vi "User Name or Public.vi"() -> ()   [LabVIEW 2020]
panel:
  out "Message":string
  in  "Use Public Profile?":bool
  in  "User Name":string
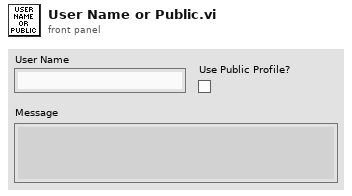
[diagram p1: front panel]
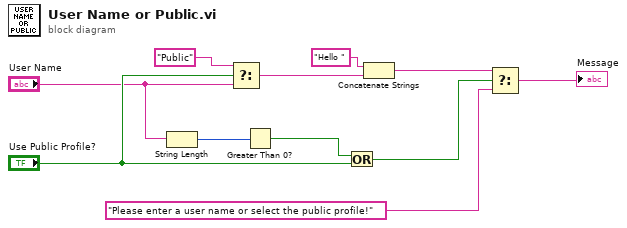
[diagram p0: block diagram]
diagram:
  n1 = String Length(string="User Name") -> (length=w11:i32)
  n2 = Select(t="Public", s="Use Public Profile?", f="User Name") -> (s? t:f=w3:string)
  n3 = Greater Than 0?(x=w11) -> (x > 0?=w10:bool)
  n4 = Or(x=w10, y="Use Public Profile?") -> (x .or. y?=w9:bool)
  n5 = Concatenate Strings "Concatenate Strings"("Hello " ("string"), w3) -> (w2:string)
  n6 = Select(t=w2, s=w9, f="Please enter a user name or select the public profile!") -> (s? t:f=→"Message":string)
